vi "EOL PMAC Clear Read History.vi"(8 "Sys Error In":errorcluster, 10 "PMAC Read History Counter":dbl, 11 "Prerun PMAC":refnum<visa-resource-name>) -> (0 "Sys Error Out":errorcluster)   [LabVIEW 2018]
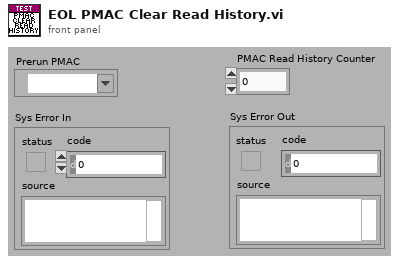
[diagram p1: front panel]
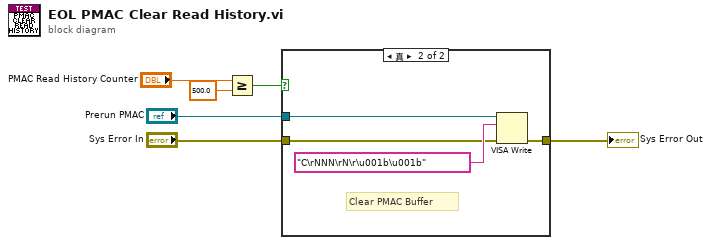
[diagram p0: block diagram]
diagram:
  n1 = Greater Or Equal?(x="PMAC Read History Counter", y=500.0) -> (x >= y?=w6:bool)
  n2 = case shown="真" w6 {
    tunnel: "Prerun PMAC" -> [_ w10]
    tunnel: [w7 w9] -> w2
    tunnel: "Sys Error In" -> [w7 w8]
    frame False {
    }
    frame True {
      # "Clear PMAC Buffer"
      n3 = VISA Write(VISA resource name=w10, write buffer="C\rNNN\rN\r\u001b\u001b", error in (no error)=w8) -> (error out=w9:errorcluster)  [unwired: 2 out]
    }
  }
  "Sys Error Out" <- w2
